vi "CheckOxideRunCheck.vi"(0 "UiDefinition":T1) -> ()   [LabVIEW 2020]
uses:
  UIReferences.ctl
  C:/Projects/RaxTagServer/LabviewDXFViewer/LabviewDXFViewer/bin/Release/LabviewDXFViewer.exe
  LabviewDXFViewer/bin/Release/LabviewDXFViewer.exe
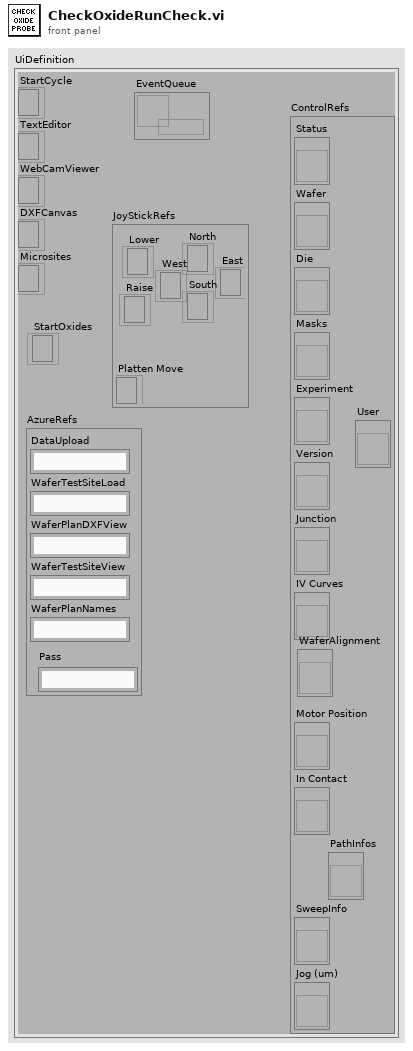
[diagram p1: front panel]
types:
  T1 = typedef "UIReferences.ctl" = cluster{"StartCycle":refnum<k24>, "TextEditor":refnum<k24>, "WebCamViewer":refnum<k24>, "DXFCanvas":refnum<k24>, "Microsites":refnum<k24>, "JoyStickRefs":cluster{"North":refnum<k24>, "Lower":refnum<k24>, "Raise":refnum<k24>, "Platten Move":refnum<k24>, "West":refnum<k24>, "East":refnum<k24>, "South":refnum<k24>}, "AzureRefs":cluster{"DataUpload":string, "WaferTestSiteLoad":string, "WaferPlanDXFView":string, "WaferTestSiteView":string, "WaferPlanNames":string, "Pass":string}, "ControlRefs":cluster{"Status":refnum<vi>, "Wafer":refnum<vi>, "Die":refnum<vi>, "Masks":refnum<vi>, "Experiment":refnum<vi>, "Version":refnum<vi>, "Junction":refnum<vi>, "IV Curves":refnum<vi>, "Motor Position":refnum<vi>, "In Contact":refnum<vi>, "SweepInfo":refnum<vi>, "Jog (um)":refnum<vi>, "PathInfos":refnum<vi>, "User":refnum<vi>, "WaferAlignment":refnum<vi>}, "EventQueue":refnum<queue>, "StartOxides":refnum<k24>}
  T2 = cluster{"Status":refnum<vi>, "Wafer":refnum<vi>, "Die":refnum<vi>, "Masks":refnum<vi>, "Experiment":refnum<vi>, "Version":refnum<vi>, "Junction":refnum<vi>, "IV Curves":refnum<vi>, "Motor Position":refnum<vi>, "In Contact":refnum<vi>, "SweepInfo":refnum<vi>, "Jog (um)":refnum<vi>, "PathInfos":refnum<vi>, "User":refnum<vi>, "WaferAlignment":refnum<vi>}
  T3 = cluster{"Die":string, "Wafer":string, "Path":path, "url":string, "Experiment":string, "Version":string, "user":string}
  T4 = typedef "WaferAlignmentType.ctl" = cluster{"Wafer Units to microns":dbl, "Rotation Misalign":dbl[], "Scale Misalign":dbl, "Steps Per micron":dbl, "Position 1":i32[], "Chip Orientation":i32, "Position 2":i32[], "Lift Distance":i32, "Position 3":i32[], "Jog Height":i32}
  T5 = cluster{"Current Range":dbl, "Source Measure Unit Channel (0: Channel A)":i32, "Waveform":waveform(dbl), "VISA resource name":refnum<visa-resource-name>, "CodeText":string}
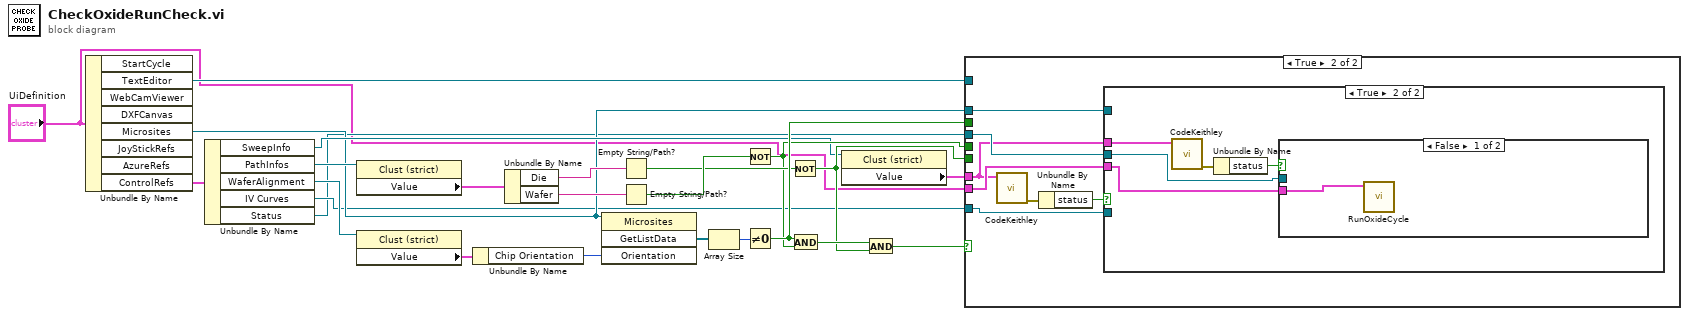
[diagram p0: block diagram]
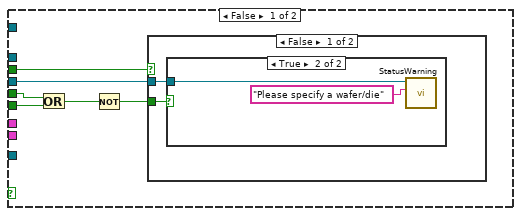
[diagram p2: hidden frame]
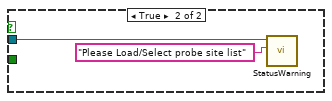
[diagram p4: hidden frame]
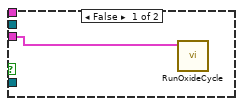
[diagram p5: hidden frame]
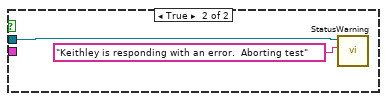
[diagram p6: hidden frame]
diagram:
  n1 = Unbundle By Name("UiDefinition") -> ("TextEditor"=w4:refnum<k24>, "Microsites"=w5:refnum<k24>, "ControlRefs"=w12:T2)  [unwired: 5 out]
  n2 = Unbundle By Name(w12) -> ("SweepInfo"=w11:refnum<vi>, "PathInfos"=w9:refnum<vi>, "WaferAlignment"=w7:refnum<vi>, "IV Curves"=w3:refnum<vi>, "Status"=w2:refnum<vi>)
  n3 = property class="Clust (strict)"(reference=w9) -> ("Value"=w8:T3)  [unwired: 1 in, 2 out]
  n4 = property class="Clust (strict)"(reference=w7) -> ("Value"=w6:T4)  [unwired: 1 in, 2 out]
  n5 = Unbundle By Name(w6) -> ("Chip Orientation"=w15:i32)
  n6 = Unbundle By Name(w8) -> ("Die"=w13:string, "Wafer"=w14:string)
  n7 = invoke class="Microsites" method="GetListData"(reference=w5, "Orientation"=w15) -> ("GetListData"=w23:refnum<k24>[])  [unwired: 2 in, 3 out]
  n8 = Empty String/Path?(string/path=w13) -> (empty?=w18:bool)
  n9 = Empty String/Path?(string/path=w14) -> (empty?=w19:bool)
  n10 = Array Size(array=w23) -> (size(s)=w24:i32)
  n11 = Not(x=w19) -> (.not. x?=w16:bool)
  n12 = Not Equal To 0?(x=w24) -> (x != 0?=w20:bool)
  n13 = Not(x=w18) -> (.not. x?=w17:bool)
  n14 = And(x=w20, y=w16) -> (x .and. y?=w22:bool)
  n15 = property class="Clust (strict)"(reference=w11) -> ("Value"=w10:T5)  [unwired: 1 in, 2 out]
  n16 = And(x=w22, y=w17) -> (x .and. y?=w21:bool)
  n17 = case shown="True" w21 {
    tunnel: w20 -> [w30 _]
    tunnel: w16 -> [w29 _]
    tunnel: w17 -> [w28 _]
    tunnel: w4 -> [_ _]
    tunnel: w5 -> [_ w43]
    tunnel: w10 -> [_ w37]
    tunnel: w3 -> [_ w42]
    tunnel: w2 -> [w25 w39]
    tunnel: "UiDefinition" -> [_ w38]
    frame False {
      n18 = Or(x=w29, y=w28) -> (x .or. y?=w27:bool)
      n19 = Not(x=w27) -> (.not. x?=w26:bool)
      n20 = case shown="False" w30 {
        tunnel: w26 -> [w32 _]
        tunnel: w25 -> [w31 w35]
        frame False {
          n21 = case shown="True" w32 {
            tunnel: w31 -> [_ w33]
            frame False {
            }
            frame True {
              n22 = call "StatusWarning.vi"("Text.Text"="Please specify a wafer/die", "String in"=w33) -> ()  [unwired: 10 in]
            }
          }
        }
        frame True {
          n23 = call "StatusWarning.vi"("Text.Text"="Please Load/Select probe site list", "String in"=w35) -> ()  [unwired: 10 in]
        }
      }
    }
    frame True {
      n24 = call "CodeKeithley.vi"("SweepInfo"=w37) -> ("error out"=w41:errorcluster)  [unwired: 10 in]
      n25 = Unbundle By Name(w41) -> ("status"=w40:bool)
      n26 = case shown="True" w40 {
        tunnel: w43 -> [_ _]
        tunnel: w42 -> [_ _]
        tunnel: w39 -> [_ w49]
        tunnel: w38 -> [w44 w45]
        tunnel: w37 -> [_ w48]
        frame False {
          n27 = call "RunOxideCycle.vi"("UiDefinition"=w44) -> ()  [unwired: 10 in]
        }
        frame True {
          n28 = call "CodeKeithley.vi"("SweepInfo"=w48) -> ("error out"=w47:errorcluster)  [unwired: 10 in]
          n29 = Unbundle By Name(w47) -> ("status"=w46:bool)
          n30 = case shown="False" w46 {
            tunnel: w49 -> [_ w51]
            tunnel: w45 -> [w50 _]
            frame False {
              n31 = call "RunOxideCycle.vi"("UiDefinition"=w50) -> ()  [unwired: 10 in]
            }
            frame True {
              n32 = call "StatusWarning.vi"("Text.Text"="Keithley is responding with an error.  Aborting test", "String in"=w51) -> ()  [unwired: 10 in]
            }
          }
        }
      }
    }
  }
